vi "Selftest Device.vi"(8 "error in (no error)":errorcluster, 10 "Self-Test":bool, 11 "CS++DeviceActor in":refnum<class "CS++DeviceActor.lvclass">) -> (0 "error out":errorcluster, 3 "CS++DeviceActor out":refnum<class "CS++DeviceActor.lvclass">)   [LabVIEW 2014, in "CS++DeviceActor.lvlib" / "CS++DeviceActor.lvclass"]
doc: "Perform device selftest."
uses:
  CS++DeviceActor.lvclass
  CS++DeviceActor.lvclass/CS++DeviceActor.ctl
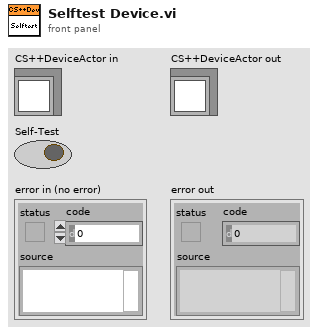
[diagram p1: front panel]
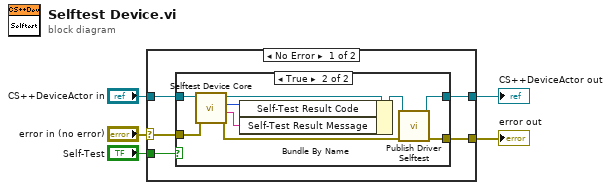
[diagram p0: block diagram]
diagram:
  n1 = case shown="No Error" "error in (no error)" {
    selector: "error in (no error)" -> [w10 w23]
    tunnel: [w8 w23] -> w4
    tunnel: [w7 w22] -> w2
    tunnel: "CS++DeviceActor in" -> [w9 w22]
    tunnel: "Self-Test" -> [w6 _]
    frame No Error {
      n2 = case shown="True" w6 {
        tunnel: w10 -> [w11 w21]
        tunnel: w9 -> [w12 w20]
        tunnel: [w11 w15] -> w8
        tunnel: [w12 w13] -> w7
        frame False {
        }
        frame True {
          n3 = call-dynamic "Selftest Device Core.vi"("error in (no error)"=w21, "CS++DeviceActor in"=w20) -> ("error out"=w16:errorcluster, "Self-Test Result Message"=w17:string, "Self-Test Result Code"=w18:i32, "CS++DeviceActor out"=w19:refnum<class "CS++DeviceActor.lvclass">)  [unwired: 6 in]
          n4 = Bundle By Name(cluster=w19, "Self-Test Result Code"=w18, "Self-Test Result Message"=w17) -> (w14:refnum<class "CS++DeviceActor.lvclass">)
          n5 = call "Publish Driver Selftest.vi"("error in (no error)"=w16, "CS++DeviceActor in"=w14) -> ("error out"=w15:errorcluster, "CS++DeviceActor out"=w13:refnum<class "CS++DeviceActor.lvclass">)  [unwired: 8 in]
        }
      }
    }
    frame Error {
    }
  }
  "error out" <- w4
  "CS++DeviceActor out" <- w2
